vi "sortItIntoArray.vi"(0 "element":u32, 1 "VoltArray":u32[](array[numeric]), 3 "actIndex":i32, 5 "CounterArray":u32[][][](array[numeric])) -> (14 "VoltArrayOut":u32[](array[numeric]), 17 "actIndexOut":i32, 19 "CounterArrayOut":u32[][][](array[numeric]))   [LabVIEW 2014]
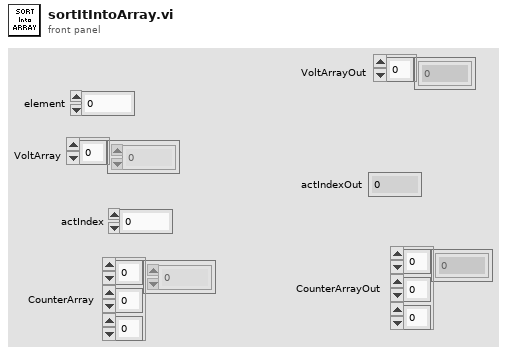
[diagram p1: front panel]
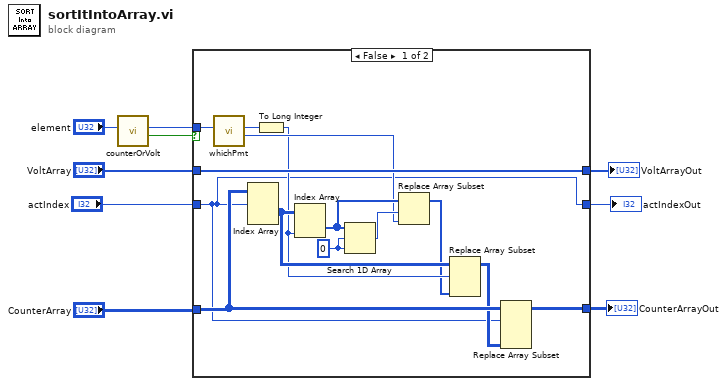
[diagram p0: block diagram]
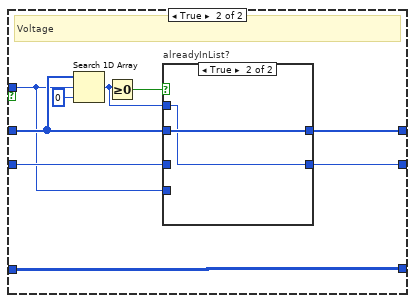
[diagram p2: hidden frame]
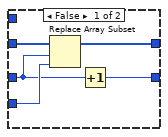
[diagram p3: hidden frame]
diagram:
  n1 = call "counterOrVolt.vi"("element"="element") -> ("volt"=w7:bool, "elementOut"=w6:u32)  [unwired: 9 in]
  n2 = case shown="False" w7 {
    tunnel: "VoltArray" -> [w23 w30]
    tunnel: w6 -> [w22 w26]
    tunnel: "actIndex" -> [w10 w27]
    tunnel: [w23 w29] -> w4
    tunnel: "CounterArray" -> [w13 w28]
    tunnel: [w11 w28] -> w2
    tunnel: [w10 w25] -> w1
    frame False {
      w20 = u32 0 ("element")
      n3 = call "whichPmt.vi"("element"=w22) -> ("elementOut"=w17:u32, "pmtNumber"=w21:u32)  [unwired: 9 in]
      n4 = Index Array(array=w13, index (dim 0)=w10) -> (element=w16:u32[][])  [unwired: 2 in]
      n5 = To Long Integer(number=w21) -> (32bit integer=w15:i32)
      n6 = Index Array(array=w16, index (col)=w15) -> (element=w19:u32[])  [unwired: 1 in]
      n7 = Search 1D Array(1D array=w19, element=w20, start index (0)=w20) -> (index of element=w18:i32)
      n8 = Replace Array Subset(array=w19, new element=w17, index=w18) -> (w14:u32[])
      n9 = Replace Array Subset(array=w16, new element=w14, index (row)=w15) -> (w12:u32[][])  [unwired: 1 in]
      n10 = Replace Array Subset(array=w13, new element=w12, index (dim 0)=w10) -> (w11:u32[][][])  [unwired: 2 in]
    }
    frame True {
      # "Voltage"
      n11 = Search 1D Array(1D array=w30, element=w26, start index (0)=0) -> (index of element=w24:i32)
      n12 = Greater Or Equal To 0?(x=w24) -> (x >= 0?=w31:bool)
      n13 = case "alreadyInList?" shown="True" w31 {
        tunnel: w30 -> [w37 w39]
        tunnel: [w36 w39] -> w29
        tunnel: w27 -> [w34 _]
        tunnel: w26 -> [w35 _]
        tunnel: [w33 w38] -> w25
        tunnel: w24 -> [_ w38]
        frame False {
          n14 = Replace Array Subset(array=w37, new element=w35, index=w34) -> (w36:u32[])
          n15 = Increment(x=w34) -> (x+1=w33:i32)
        }
        frame True {
        }
      }
    }
  }
  "VoltArrayOut" <- w4
  "CounterArrayOut" <- w2
  "actIndexOut" <- w1
